vi "Read_raw_meas_setup.vi"(8 "Setup file string":string) -> (0 "No of Blocks":i32=1, 1 "Sampling freq (Hz)":dbl=100.0, 2 "No of samples":i32=500 min=0 step=1, 3 "Analysis Info cluster 2":T1[](array[typedef])=[{"Colour"=0, "Inst type"=enum."Pitot-static tube", "Inst name"="Manometer voltage", "Symbol"="U", "Code name"="", "Extra Info"="U", "Inst Array"=enum."PWA", "Extra Titles"=[], "Extra Values"=[], "U"=0.0, "u^2"=0.0, "u^3"=0.0, "u^4"=0.0, "Skew_u"=0.0, "Kurt_u"=0.0, "Sd Error in Mean"=0.0, "% u'/U"=0.0, "X"=0.0, "Y"=0.0, "Z"=0.0, "Timescale integral to 25%"=0.0, "Sd Error in Variance"=0.0, "Calib File"=path "", "Calib Constants"=[], "Output Position"=FALSE, "Full Stats"=FALSE, "Av Sampling Rate"=0.0, "Av No of Samples"=0.0, "Total Meas Time (s)"=0.0, "ADAM Ch Name"=""}, {"Colour"=0, "Inst type"=enum."Pitot-static tube", "Inst name"="Manometer voltage", "Symbol"="U", "Code name"="", "Extra Info"="U", "Inst Array"=enum."PWA", "Extra Titles"=[], "Extra Values"=[], "U"=0.0, "u^2"=0.0, "u^3"=0.0, "u^4"=0.0, "Skew_u"=0.0, "Kurt_u"=0.0, "Sd Error in Mean"=0.0, "% u'/U"=0.0, "X"=0.0, "Y"=0.0, "Z"=0.0, "Timescale integral to 25%"=0.0, "Sd Error in Variance"=0.0, "Calib File"=path "", "Calib Constants"=[], "Output Position"=FALSE, "Full Stats"=FALSE, "Av Sampling Rate"=0.0, "Av No of Samples"=0.0, "Total Meas Time (s)"=0.0, "ADAM Ch Name"=""}, {"Colour"=0, "Inst type"=enum."Pitot-static tube", "Inst name"="Manometer voltage", "Symbol"="U", "Code name"="", "Extra Info"="U", "Inst Array"=enum."PWA", "Extra Titles"=[], "Extra Values"=[], "U"=0.0, "u^2"=0.0, "u^3"=0.0, "u^4"=0.0, "Skew_u"=0.0, "Kurt_u"=0.0, "Sd Error in Mean"=0.0, "% u'/U"=0.0, "X"=0.0, "Y"=0.0, "Z"=0.0, "Timescale integral to 25%"=0.0, "Sd Error in Variance"=0.0, "Calib File"=path "", "Calib Constants"=[], "Output Position"=FALSE, "Full Stats"=FALSE, "Av Sampling Rate"=0.0, "Av No of Samples"=0.0, "Total Meas Time (s)"=0.0, "ADAM Ch Name"=""}, {"Colour"=0, "Inst type"=enum."Pitot-static tube", "Inst name"="Manometer voltage", "Symbol"="U", "Code name"="", "Extra Info"="U", "Inst Array"=enum."PWA", "Extra Titles"=[], "Extra Values"=[], "U"=0.0, "u^2"=0.0, "u^3"=0.0, "u^4"=0.0, "Skew_u"=0.0, "Kurt_u"=0.0, "Sd Error in Mean"=0.0, "% u'/U"=0.0, "X"=0.0, "Y"=0.0, "Z"=0.0, "Timescale integral to 25%"=0.0, "Sd Error in Variance"=0.0, "Calib File"=path "", "Calib Constants"=[], "Output Position"=FALSE, "Full Stats"=FALSE, "Av Sampling Rate"=0.0, "Av No of Samples"=0.0, "Total Meas Time (s)"=0.0, "ADAM Ch Name"=""}] {"Sd Error in Variance" format="%.2f"; "Skew_u" format="%.2f"; "% u'/U" format="%.2f"; "Sd Error in Mean" format="%.2f"; "Kurt_u" format="%.2f"; "u^4" format="%.2f"; "u^3" format="%.2f"; "U" format="%.2f"; "u^2" format="%.2f"}, 5 "Correlate?":T4(ring))   [LabVIEW 2012]
uses:
  Controls/Analysis_info_cluster.ctl
  Controls/Inst_type.ctl
  Controls/Instrument_Array.ctl
  Globals/Meas_global.vi
  Globals/LDA_meas_global_1.vi
  Globals/LDA_meas_global_2.vi
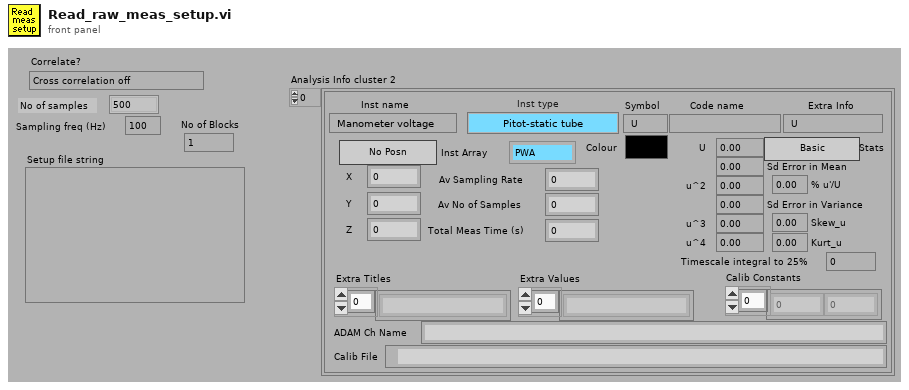
[diagram p1: front panel]
types:
  T1 = typedef "Analysis_info_cluster.ctl" = cluster{"Colour":u32, "Inst type":T2, "Inst name":string, "Symbol":string, "Code name":string, "Extra Info":string, "Inst Array":T3, "Extra Titles":string[], "Extra Values":string[], "U":dbl, "u^2":dbl, "u^3":dbl, "u^4":dbl, "Skew_u":dbl, "Kurt_u":dbl, "Sd Error in Mean":dbl, "% u'/U":dbl, "X":dbl, "Y":dbl, "Z":dbl, "Timescale integral to 25%":dbl, "Sd Error in Variance":dbl, "Calib File":path, "Calib Constants":dbl[], "Output Position":bool, "Full Stats":bool, "Av Sampling Rate":dbl, "Av No of Samples":dbl, "Total Meas Time (s)":dbl, "ADAM Ch Name":string}
  T2 = typedef "Inst_type.ctl" = enum16{"Propeller anemometer", "Raw voltage", "Pressure Transducer", "Pitot-static tube", "Preston tube", "Hot wire", "Cross wire 1", "Cross wire 2", "Generic Linear", "Generic Polynomial", "Generic BackPoly", "Fast FID", "Thermocouple", "Cold wire", "Pulsed Wire", "LDA Vel", "LDA Tran time", "LDA Arr time"}
  T3 = typedef "Instrument_Array.ctl" = enum16{"PWA", "LDA", "Analogue"}
  T4 = enum16{"Cross correlation off", "Show correlation panel", "Correlate without activating panel"}
  T5 = typedef "Post_Process.ctl" = enum16{"Take New Data", "Post Process Raw Data File"}
  T6 = enum16{"From String to Cluster", "From Cluster to String"}
  T7 = typedef "BSA_Type.ctl" = enum16{"57N11", "BSA F60"}
  T8 = typedef "LDA_Setup.ctl" = cluster{"dimensions":enum16{"1D", "2D"}, "Analogue Freq Multiplier":dbl}
  T9 = typedef "BSA_info_Cluster.ctl" = cluster{"GPIB Address":string, "No of Check Bytes":i32, "Extra Info":string, "COLOUR":u32, "Wavelength (nm)":dbl}
  T10 = typedef "Graph_Type.ctl" = enum16{"Show no graph", "Voltage trace", "Velocity trace", "Vel histogram", "Spectrum", "f.E(f) v Log f", "Auto-Corr"}
  T11 = cluster{"Plot 1":u16, "Plot 2":u16, "Save graph":u16, "Plot Type":T10}
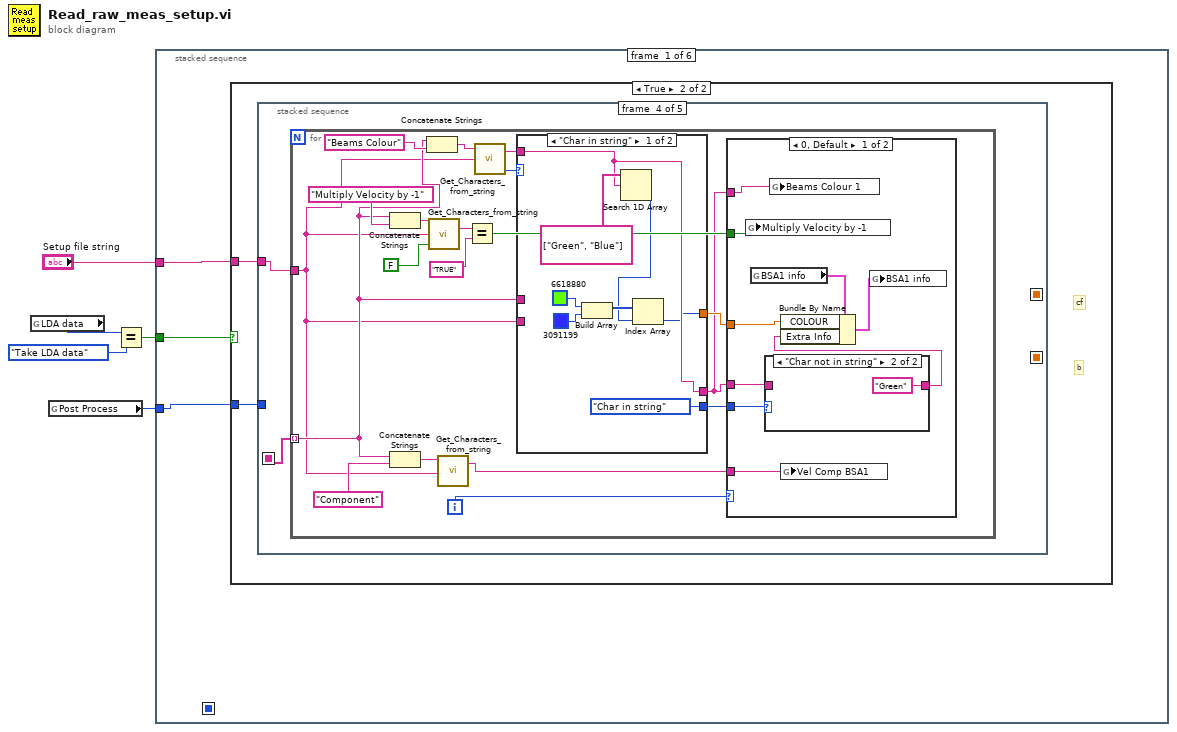
[diagram p0: block diagram]
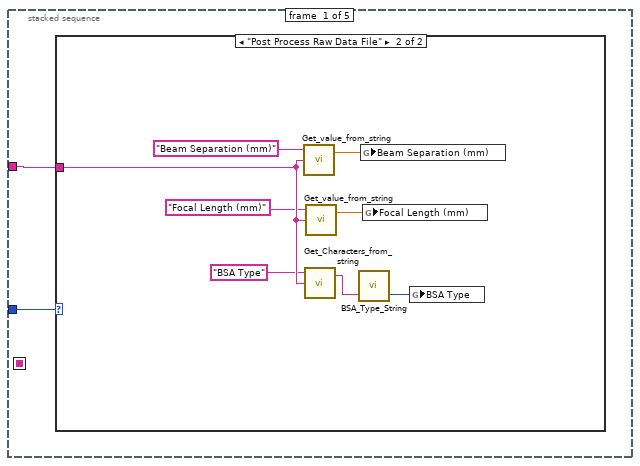
[diagram p3: hidden frame]
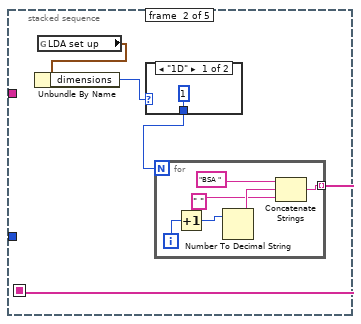
[diagram p5: hidden frame]
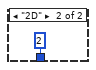
[diagram p6: hidden frame]
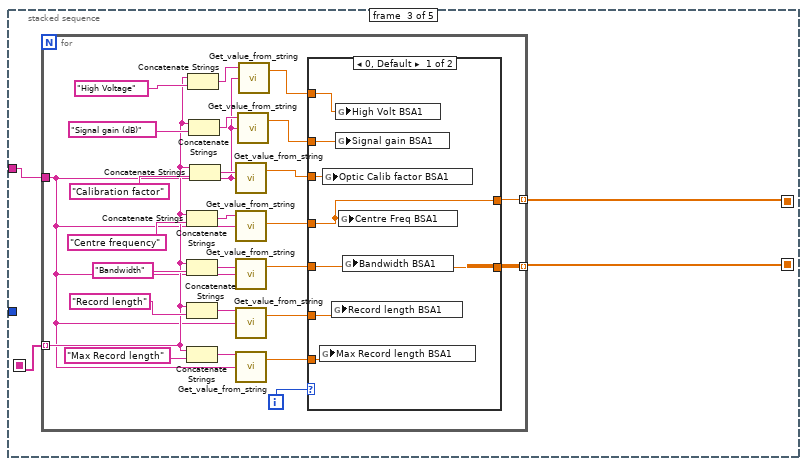
[diagram p7: hidden frame]
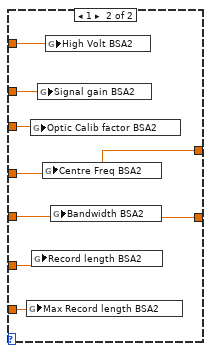
[diagram p8: hidden frame]
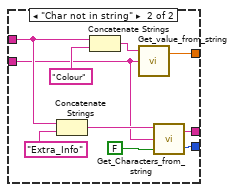
[diagram p9: hidden frame]
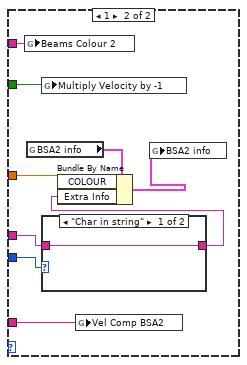
[diagram p11: hidden frame]
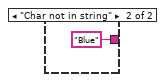
[diagram p12: hidden frame]
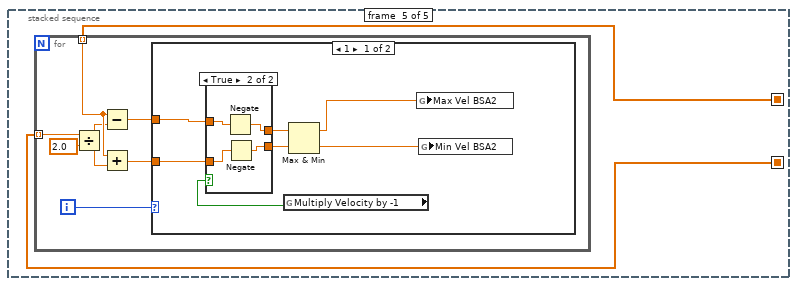
[diagram p13: hidden frame]
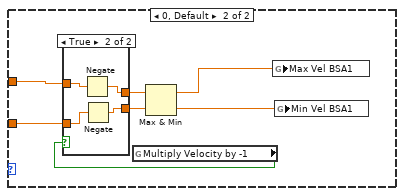
[diagram p15: hidden frame]
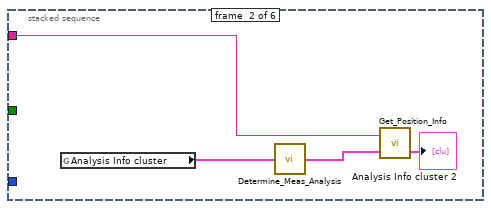
[diagram p17: hidden frame]
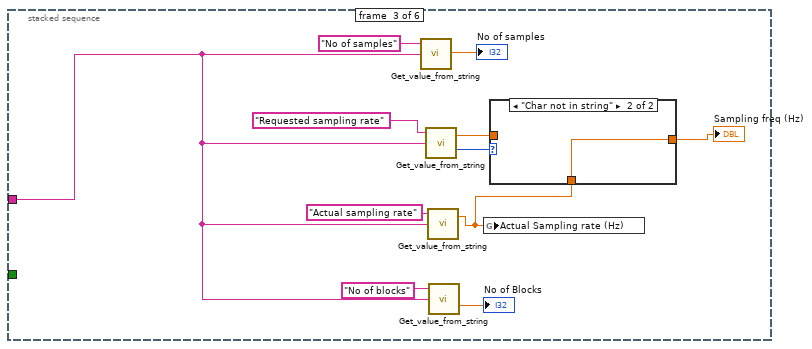
[diagram p18: hidden frame]
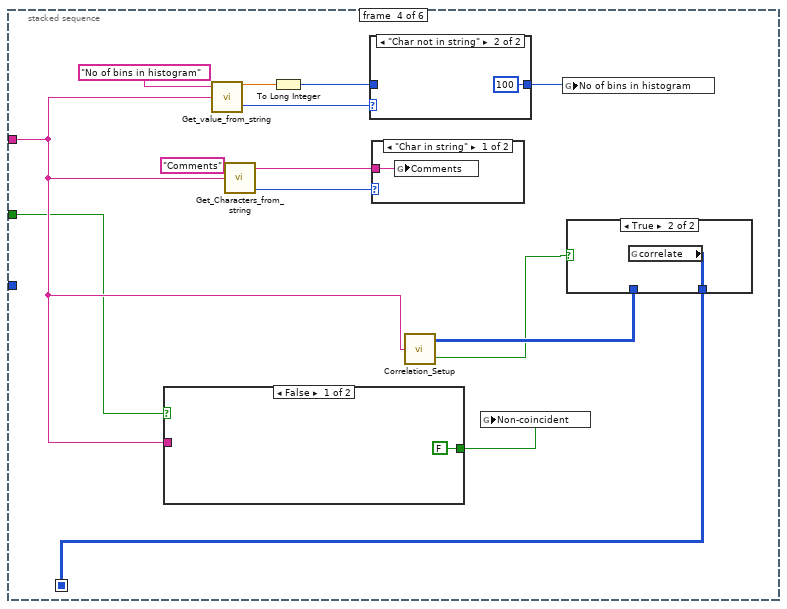
[diagram p20: hidden frame]
diagram:
  n1 = global read "Meas_global.vi" "LDA data"() -> (w3:enum16{"No LDA data", "Take LDA data"})
  n2 = global read "Meas_global.vi" "Post Process"() -> (w5:T5)
  n3 = Equal?(x=w3, y=enum16{"No LDA data", "Take LDA data"}."Take LDA data" ("LDA data")) -> (x = y?=w2:bool)
  n4 = stacked-sequence {
    seq-local: [_ _ _ w195 _ _] -> [_ _ _ _ w220 _]
    tunnel: w5 -> [w6 _ _ _ _ _]
    tunnel: w2 -> [w8 _ _ w190 _ _]
    tunnel: "Setup file string" -> [w7 w176 w182 w191 _ w223]
    frame #0 {
      n5 = case shown="True" w8 {
        tunnel: w7 -> [_ w10]
        tunnel: w6 -> [_ w9]
        frame False {
        }
        frame True {
          # "b"
          # "cf"
          n6 = stacked-sequence {
            seq-local: [_ w23 _ _ _] -> [_ _ w35 w77 _]
            seq-local: [_ _ w33 _ _] -> [_ _ _ _ w138]
            seq-local: [_ _ w34 _ _] -> [_ _ _ _ w139]
            tunnel: w10 -> [w11 _ w36 w78 _]
            tunnel: w9 -> [w12 _ _ _ _]
            frame #0 {
              n7 = case shown="\"Post Process Raw Data File\"" w12 {
                tunnel: w11 -> [_ w20]
                frame "Take New Data" {
                }
                frame "Post Process Raw Data File" {
                  n8 = call "Get_value_from_string.vi"("Input string"=w20, "Variable name"="Beam Separation (mm)" ("Label for characters")) -> ("Value"=w13:dbl)  [unwired: 1 in, 1 out]
                  n9 = call "Get_Characters_from_string.vi"("Input string"=w20, "Variable name"="BSA Type" ("Label for characters")) -> ("Value"=w16:string)  [unwired: 1 in, 1 out]
                  n10 = call "Get_value_from_string.vi"("Input string"=w20, "Variable name"="Focal Length (mm)" ("Label for characters")) -> ("Value"=w14:dbl)  [unwired: 1 in, 1 out]
                  n11 = call "BSA_Type_String.vi"("BSA String in"=w16) -> ("BSA Type Out"=w15:T7)  [unwired: 1 in, 1 out]
                  n12 = global write "LDA_meas_global_1.vi" "Beam Separation (mm)"(w13) -> ()
                  n13 = global write "LDA_meas_global_1.vi" "Focal Length (mm)"(w14) -> ()
                  n14 = global write "LDA_meas_global_1.vi" "BSA Type"(w15) -> ()
                }
              }
            }
            frame #1 {
              n15 = global read "Meas_global.vi" "LDA set up"() -> (w22:T8)
              n16 = Unbundle By Name(w22) -> ("dimensions"=w21:enum16{"1D", "2D"})
              n17 = case shown="\"1D\"" w21 {
                tunnel: [1 2] -> w24
                frame "1D" {
                }
                frame "2D" {
                }
              }
              n18 = for {
                N: w24 -> [_]
                tunnel: [w26] -> w23 mode=indexing
                i -> [w28]
                n19 = Increment(x=w28) -> (x+1=w27:i32)
                n20 = Number To Decimal String(number=w27) -> (decimal integer string=w30:string)  [unwired: 1 out]
                n21 = Concatenate Strings("BSA ", w30, " ") -> (w26:string)
              }
            }
            frame #2 {
              n22 = for {
                tunnel: w36 -> [w37]
                tunnel: w35 -> [w38] mode=indexing
                tunnel: [w50] -> w34 mode=indexing
                tunnel: [w49] -> w33 mode=indexing
                i -> [w54]
                n23 = Concatenate Strings(w38, "Centre frequency") -> (w57:string)
                n24 = Concatenate Strings(w38, "Bandwidth") -> (w56:string)
                n25 = Concatenate Strings(w38, "Record length") -> (w55:string)
                n26 = Concatenate Strings(w38, "Max Record length") -> (w40:string)
                n27 = Concatenate Strings(w38, "High Voltage") -> (w44:string)
                n28 = Concatenate Strings(w38, "Signal gain (dB)") -> (w45:string)
                n29 = Concatenate Strings(w38, "Calibration factor") -> (w58:string)
                n30 = call "Get_value_from_string.vi"("Input string"=w37, "Variable name"=w58) -> ("Value"=w48:dbl)  [unwired: 1 in, 1 out]
                n31 = call "Get_value_from_string.vi"("Input string"=w37, "Variable name"=w57) -> ("Value"=w53:dbl)  [unwired: 1 in, 1 out]
                n32 = call "Get_value_from_string.vi"("Input string"=w37, "Variable name"=w56) -> ("Value"=w52:dbl)  [unwired: 1 in, 1 out]
                n33 = call "Get_value_from_string.vi"("Input string"=w37, "Variable name"=w55) -> ("Value"=w51:dbl)  [unwired: 1 in, 1 out]
                n34 = call "Get_value_from_string.vi"("Input string"=w37, "Variable name"=w40) -> ("Value"=w41:dbl)  [unwired: 1 in, 1 out]
                n35 = call "Get_value_from_string.vi"("Input string"=w37, "Variable name"=w45) -> ("Value"=w43:dbl)  [unwired: 1 in, 1 out]
                n36 = call "Get_value_from_string.vi"("Input string"=w37, "Variable name"=w44) -> ("Value"=w42:dbl)  [unwired: 1 in, 1 out]
                n37 = case shown="0, Default" w54 {
                  tunnel: w53 -> [w66 w74]
                  tunnel: w52 -> [w67 w73]
                  tunnel: w51 -> [w68 w76]
                  tunnel: w48 -> [w69 w75]
                  tunnel: [w67 w73] -> w50
                  tunnel: [w66 w74] -> w49
                  tunnel: w43 -> [w65 w71]
                  tunnel: w42 -> [w64 w72]
                  tunnel: w41 -> [w63 w70]
                  frame 0, Default {
                    n38 = global write "LDA_meas_global_1.vi" "Max Record length BSA1"(w63) -> ()
                    n39 = global write "LDA_meas_global_1.vi" "Optic Calib factor BSA1"(w69) -> ()
                    n40 = global write "LDA_meas_global_1.vi" "Record length BSA1"(w68) -> ()
                    n41 = global write "LDA_meas_global_1.vi" "High Volt BSA1"(w64) -> ()
                    n42 = global write "LDA_meas_global_1.vi" "Signal gain BSA1"(w65) -> ()
                    n43 = global write "LDA_meas_global_1.vi" "Centre Freq BSA1"(w66) -> ()
                    n44 = global write "LDA_meas_global_1.vi" "Bandwidth BSA1"(w67) -> ()
                  }
                  frame 1 {
                    n45 = global write "LDA_meas_global_2.vi" "Max Record length BSA2"(w70) -> ()
                    n46 = global write "LDA_meas_global_2.vi" "Optic Calib factor BSA2"(w75) -> ()
                    n47 = global write "LDA_meas_global_2.vi" "Record length BSA2"(w76) -> ()
                    n48 = global write "LDA_meas_global_2.vi" "Signal gain BSA2"(w71) -> ()
                    n49 = global write "LDA_meas_global_2.vi" "Centre Freq BSA2"(w74) -> ()
                    n50 = global write "LDA_meas_global_2.vi" "High Volt BSA2"(w72) -> ()
                    n51 = global write "LDA_meas_global_2.vi" "Bandwidth BSA2"(w73) -> ()
                  }
                }
              }
            }
            frame #3 {
              n52 = for {
                tunnel: w78 -> [w82]
                tunnel: w77 -> [w83] mode=indexing
                i -> [w96]
                n53 = Concatenate Strings(w83, "Multiply Velocity by -1") -> (w93:string)
                n54 = Concatenate Strings(w83, "Component") -> (w97:string)
                n55 = Concatenate Strings(w83, "Beams Colour") -> (w86:string)
                n56 = call "Get_Characters_from_string.vi"("Show Dialog?"=FALSE, "Input string"=w82, "Variable name"=w93) -> ("Value"=w91:string)  [unwired: 1 out]
                n57 = call "Get_Characters_from_string.vi"("Input string"=w82, "Variable name"=w97) -> ("Value"=w94:string)  [unwired: 1 in, 1 out]
                n58 = Equal?(x=w91, y="TRUE") -> (x = y?=w89:bool)
                n59 = call "Get_Characters_from_string.vi"("Input string"=w82, "Variable name"=w86) -> ("Status"=w81:enum16{"Char in string", "Char not in string"}, "Value"=w80:string)  [unwired: 1 in]
                n60 = case shown="\"Char in string\"" w81 {
                  tunnel: [enum16{"Char in string", "Char not in string"}."Char in string" ("Status") w112] -> w88
                  tunnel: [w98 w111] -> w84
                  tunnel: [w100 w108] -> w79
                  tunnel: w83 -> [_ w107]
                  tunnel: w82 -> [_ w106]
                  tunnel: w80 -> [w100 _]
                  frame "Char in string" {
                    n61 = Build Array(u32 6618880, u32 3091199) -> (w102:u32[])
                    n62 = Search 1D Array(1D array=string[] ["Green", "Blue"], element=w100) -> (index of element=w101:i32)  [unwired: 1 in]
                    n63 = Index Array(array=w102, index=w101) -> (element=w98:u32)
                  }
                  frame "Char not in string" {
                    n64 = Concatenate Strings(w107, "Extra_Info" ("string")) -> (w115:string)
                    n65 = Concatenate Strings(w107, "Colour") -> (w109:string)
                    n66 = call "Get_value_from_string.vi"("Input string"=w106, "Variable name"=w109) -> ("Value"=w111:dbl)  [unwired: 1 in, 1 out]
                    n67 = call "Get_Characters_from_string.vi"("Show Dialog?"=FALSE, "Input string"=w106, "Variable name"=w115) -> ("Status"=w112:enum16{"Char in string", "Char not in string"}, "Value"=w108:string)
                  }
                }
                n68 = case shown="0, Default" w96 {
                  tunnel: w84 -> [w123 w134]
                  tunnel: w94 -> [w122 w133]
                  tunnel: w89 -> [w121 w132]
                  tunnel: w88 -> [w120 w129]
                  tunnel: w79 -> [w119 w130]
                  tunnel: w79 -> [w116 w127]
                  frame 0, Default {
                    n69 = global write "LDA_meas_global_1.vi" "Multiply Velocity by -1"(w121) -> ()
                    n70 = global read "LDA_meas_global_1.vi" "BSA1 info"() -> (w124:T9)
                    n71 = case shown="\"Char not in string\"" w120 {
                      tunnel: w119 -> [w125 _]
                      tunnel: [w125 "Green" ("Value")] -> w117
                      frame "Char in string" {
                      }
                      frame "Char not in string" {
                      }
                    }
                    n72 = global write "LDA_meas_global_1.vi" "Beams Colour 1"(w116) -> ()
                    n73 = Bundle By Name(cluster=w124, "COLOUR"=w123, "Extra Info"=w117) -> (w118:T9)
                    n74 = global write "LDA_meas_global_1.vi" "Vel Comp BSA1"(w122) -> ()
                    n75 = global write "LDA_meas_global_1.vi" "BSA1 info"(w118) -> ()
                  }
                  frame 1 {
                    n76 = global write "LDA_meas_global_2.vi" "Beams Colour 2"(w127) -> ()
                    n77 = global read "LDA_meas_global_2.vi" "BSA2 info"() -> (w135:T9)
                    n78 = global write "LDA_meas_global_2.vi" "Multiply Velocity by -1"(w132) -> ()
                    n79 = case shown="\"Char in string\"" w129 {
                      tunnel: w130 -> [w136 _]
                      tunnel: [w136 "Blue" ("Value")] -> w128
                      frame "Char in string" {
                      }
                      frame "Char not in string" {
                      }
                    }
                    n80 = Bundle By Name(cluster=w135, "COLOUR"=w134, "Extra Info"=w128) -> (w131:T9)
                    n81 = global write "LDA_meas_global_2.vi" "Vel Comp BSA2"(w133) -> ()
                    n82 = global write "LDA_meas_global_2.vi" "BSA2 info"(w131) -> ()
                  }
                }
              }
            }
            frame #4 {
              n83 = for {
                tunnel: w139 -> [w145] mode=indexing
                tunnel: w138 -> [w144] mode=indexing
                i -> [w140]
                n84 = Divide(x=w145, y=2.0) -> (x/y=w143:dbl)
                n85 = Subtract(x=w144, y=w143) -> (x-y=w141:dbl)
                n86 = Add(x=w144, y=w143) -> (x+y=w142:dbl)
                n87 = case shown="1" w140 {
                  tunnel: w142 -> [w153 w166]
                  tunnel: w141 -> [w152 w165]
                  frame 1 {
                    n88 = global read "LDA_meas_global_2.vi" "Multiply Velocity by -1"() -> (w149:bool)
                    n89 = case shown="True" w149 {
                      tunnel: w153 -> [w154 w159]
                      tunnel: w152 -> [w155 w158]
                      tunnel: [w155 w157] -> w151
                      tunnel: [w154 w156] -> w150
                      frame False {
                      }
                      frame True {
                        n90 = Negate(x=w158) -> (-x=w157:dbl)
                        n91 = Negate(x=w159) -> (-x=w156:dbl)
                      }
                    }
                    n92 = Max & Min(x=w151, y=w150) -> (max(x,y)=w147:dbl, min(x,y)=w148:dbl)
                    n93 = global write "LDA_meas_global_2.vi" "Max Vel BSA2"(w147) -> ()
                    n94 = global write "LDA_meas_global_2.vi" "Min Vel BSA2"(w148) -> ()
                  }
                  frame 0, Default {
                    n95 = global read "LDA_meas_global_1.vi" "Multiply Velocity by -1"() -> (w162:bool)
                    n96 = case shown="True" w162 {
                      tunnel: w166 -> [w167 w172]
                      tunnel: w165 -> [w168 w171]
                      tunnel: [w168 w170] -> w164
                      tunnel: [w167 w169] -> w163
                      frame False {
                      }
                      frame True {
                        n97 = Negate(x=w171) -> (-x=w170:dbl)
                        n98 = Negate(x=w172) -> (-x=w169:dbl)
                      }
                    }
                    n99 = Max & Min(x=w164, y=w163) -> (max(x,y)=w160:dbl, min(x,y)=w161:dbl)
                    n100 = global write "LDA_meas_global_1.vi" "Max Vel BSA1"(w160) -> ()
                    n101 = global write "LDA_meas_global_1.vi" "Min Vel BSA1"(w161) -> ()
                  }
                }
              }
            }
          }
        }
      }
    }
    frame #1 {
      n102 = global read "Meas_global.vi" "Analysis Info cluster"() -> (w174:T1[])
      n103 = call "Determine_Meas_Analysis.vi"("Analysis info Cluster In"=w174) -> ("Analysis info Cluster Out"=w173:T1[])
      n104 = call "Get_Position_Info.vi"("Analysis Info cluster"=w173, "Setup file string"=w176) -> ("Analysis Info cluster 2"=→"Analysis Info cluster 2":T1[])  [unwired: 1 in]
    }
    frame #2 {
      n105 = call "Get_value_from_string.vi"("Input string"=w182, "Variable name"="No of samples") -> ("Value"=→"No of samples":dbl)  [unwired: 1 in, 1 out]
      n106 = call "Get_value_from_string.vi"("Input string"=w182, "Variable name"="Requested sampling rate") -> ("Status"=w180:enum16{"Char in string", "Char not in string"}, "Value"=w178:dbl)  [unwired: 1 in]
      n107 = call "Get_value_from_string.vi"("Input string"=w182, "Variable name"="Actual sampling rate") -> ("Value"=w177:dbl)  [unwired: 1 in, 1 out]
      n108 = call "Get_value_from_string.vi"("Input string"=w182, "Variable name"="No of blocks") -> ("Value"=→"No of Blocks":dbl)  [unwired: 1 in, 1 out]
      n109 = global write "Meas_global.vi" "Actual Sampling rate (Hz)"(w177) -> ()
      n110 = case shown="\"Char not in string\"" w180 {
        tunnel: [w188 w189] -> w179
        tunnel: w178 -> [w188 _]
        tunnel: w177 -> [_ w189]
        frame "Char in string" {
        }
        frame "Char not in string" {
        }
      }
      "Sampling freq (Hz)" <- w179
    }
    frame #3 {
      n111 = case shown="False" w190 {
        tunnel: [FALSE w206] -> w192
        tunnel: w191 -> [_ w205]
        frame False {
        }
        frame True {
          n112 = call "Get_Characters_from_string.vi"("Input string"=w205, "Variable name"="Non-Coincident Mode" ("Pre Setup String")) -> ("Value"=w208:string)  [unwired: 1 in, 1 out]
          n113 = Equal?(x=w208, y="TRUE") -> (x = y?=w206:bool)
        }
      }
      n114 = call "Get_value_from_string.vi"("Input string"=w191, "Variable name"="No of bins in histogram") -> ("Status"=w202:enum16{"Char in string", "Char not in string"}, "Value"=w201:dbl)  [unwired: 1 in]
      n115 = call "Get_Characters_from_string.vi"("Input string"=w191, "Variable name"="Comments") -> ("Status"=w199:enum16{"Char in string", "Char not in string"}, "Value"=w198:string)  [unwired: 1 in]
      n116 = To Long Integer(number=w201) -> (32bit integer=w200:i32)
      n117 = case shown="\"Char not in string\"" w202 {
        tunnel: w200 -> [w213 _]
        tunnel: [w213 100] -> w196
        frame "Char in string" {
        }
        frame "Char not in string" {
        }
      }
      n118 = case shown="\"Char in string\"" w199 {
        tunnel: w198 -> [w212 _]
        frame "Char in string" {
          n119 = global write "Meas_global.vi" "Comments"(w212) -> ()
        }
        frame "Char not in string" {
        }
      }
      n120 = call "Correlation_Setup.vi"("Input string"=w191) -> ("Correlate"=w194:i32[][], "Error?"=w193:bool)
      n121 = global write "LDA_meas_global_1.vi" "Non-coincident"(w192) -> ()
      n122 = global write "Meas_global.vi" "No of bins in histogram"(w196) -> ()
      n123 = case shown="True" w193 {
        tunnel: w194 -> [w210 _]
        tunnel: [w210 w211] -> w195
        frame False {
          n124 = global write "Meas_global.vi" "correlate"(w210) -> ()
        }
        frame True {
          n125 = global read "Meas_global.vi" "correlate"() -> (w211:i32[][])
        }
      }
    }
    frame #4 {
      n126 = Array Size(array=w220) -> (size(s)=w222:i32[])
      n127 = Index Array(array=w222, index=0) -> (element=w219:i32)
      n128 = Equal To 0?(x=w219) -> (x = 0?=w215:bool)
      n129 = Select(t=T4."Cross correlation off" ("Correlate?"), s=w215, f=T4."Correlate without activating panel" ("Correlate?")) -> (s? t:f=→"Correlate?":T4)
    }
    frame #5 {
      n130 = call "Save_Load_Graph_Setup.vi"("Setup String in"=w223, "Graph Number"=1, "Mode"=T6."From String to Cluster") -> ("Variables found?"=w229:bool, "Graph Out"=w228:T11)  [unwired: 1 in, 1 out]
      n131 = call "Save_Load_Graph_Setup.vi"("Setup String in"=w223, "Graph Number"=2, "Mode"=T6."From String to Cluster") -> ("Variables found?"=w225:bool, "Graph Out"=w224:T11)  [unwired: 1 in, 1 out]
      n132 = case shown="True" w229 {
        tunnel: w228 -> [_ w233]
        frame False {
        }
        frame True {
          n133 = global write "Meas_global.vi" "First Graph"(w233) -> ()
        }
      }
      n134 = case shown="True" w225 {
        tunnel: w224 -> [_ w232]
        frame False {
        }
        frame True {
          n135 = global write "Meas_global.vi" "Second Graph"(w232) -> ()
        }
      }
    }
  }
